vi "RSZVB Get Port Waveguide Attenuator Type.vi"(8 "error in (no error)":errorcluster {"code" format="%.0x"}, 9 "Port (1)":i32=1, 10 "Channel (1)":i32=1, 11 "VISA session":refnum<visa-resource-name>) -> (0 "error out":errorcluster {"code" format="%.0x"}, 2 "Waveguide Attenuator":i32, 3 "dup VISA session":refnum<visa-resource-name>)   [LabVIEW 2011]
doc: "This VI returns the waveguide attenuator type of the converter port <Pt> and attenuation for a converter with electronic or mechanical attenuators at port <Pt>.\n\nRemote-control command(s):\nSOURce<Ch>:POWer<Pt>:CONVerter:TRANsfer:ATTenuator?"
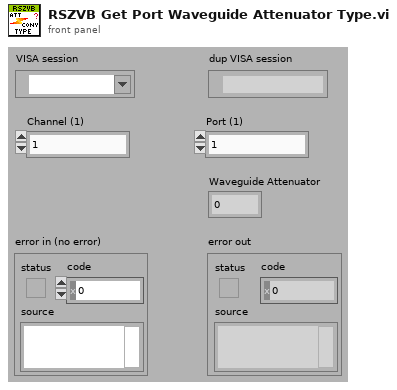
[diagram p1: front panel]
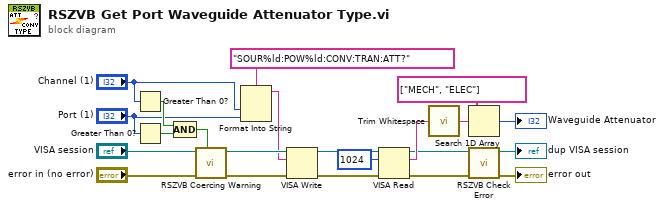
[diagram p0: block diagram]
diagram:
  n1 = Greater Than 0?(x="Channel (1)") -> (x > 0?=w18:bool)
  n2 = Greater Than 0?(x="Port (1)") -> (x > 0?=w17:bool)
  n3 = Compound Arithmetic op=AND(w18, w17) -> (w19:bool)
  n4 = call "RSZVB Coercing Warning.vi"("In Range?"=w19, "error in (no error)"="error in (no error)", "VISA session"="VISA session") -> ("error out"=w20:errorcluster, "dup VISA session"=w21:refnum<visa-resource-name>)  [unwired: 7 in]
  n5 = Format Into String(format string="SOUR%ld:POW%ld:CONV:TRAN:ATT?", "Channel (1)", "Port (1)") -> (resulting string=w12:string)  [unwired: 2 in, 1 out]
  n6 = VISA Write(VISA resource name=w21, write buffer=w12, error in (no error)=w20) -> (VISA resource name out=w4:refnum<visa-resource-name>, error out=w5:errorcluster)  [unwired: 1 out]
  n7 = VISA Read(VISA resource name=w4, byte count=u32 1024, error in (no error)=w5) -> (VISA resource name out=w7:refnum<visa-resource-name>, read buffer=w10:string, error out=w8:errorcluster)  [unwired: 1 out]
  n8 = call <vilib>:"Trim Whitespace.vi"("string"=w10) -> ("trimmed string"=w9:string)  [unwired: 1 in]
  n9 = Search 1D Array(1D array=string[] ["MECH", "ELEC"], element=w9) -> (index of element=→"Waveguide Attenuator":i32)  [unwired: 1 in]
  n10 = call "RSZVB Check Error.vi"("error in (no error)"=w8, "VISA session"=w7) -> ("error out"=→"error out":errorcluster, "dup VISA session"=→"dup VISA session":refnum<visa-resource-name>)  [unwired: 8 in]
